vi "Main_FGV_Time.vi"(7 "Time Action":enum16{"Start", "Read", "Clear"}(ring)) -> (3 "Time":u32)   [LabVIEW 2015]
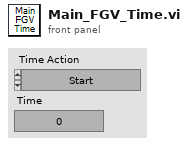
[diagram p1: front panel]
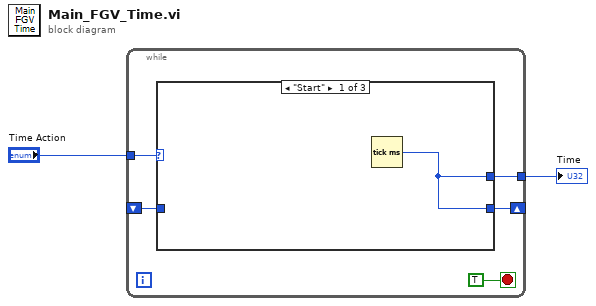
[diagram p0: block diagram]
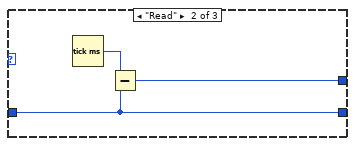
[diagram p2: hidden frame]
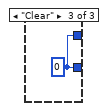
[diagram p3: hidden frame]
diagram:
  n1 = while {
    tunnel: "Time Action" -> [w6]
    shift-right: [w5] -> _
    shift-left: _ -> [w4]
    tunnel: [w3] -> w1
    stop <- TRUE stop-if-true
    n2 = case shown="\"Start\"" w6 {
      tunnel: [w8 w10 w12] -> w5
      tunnel: w4 -> [_ w10 _]
      tunnel: [w8 w9 w12] -> w3
      frame "Start" {
        n3 = Tick Count (ms)() -> (millisecond timer value=w8:u32)
      }
      frame "Read" {
        n4 = Tick Count (ms)() -> (millisecond timer value=w11:u32)
        n5 = Subtract(x=w11, y=w10) -> (x-y=w9:u32)
      }
      frame "Clear" {
        w12 = u32 0 ("millisecond timer value")
      }
    }
  }
  "Time" <- w1
